vi "Que_Build Initialize Command Set.vi"(8 "Error":errorcluster, 11 "Icon Source Is From A VI":bool) -> (0 "Error Out":errorcluster, 3 "Command Set Out":T1[](array[typedef]))   [LabVIEW 2009]
doc: "Builds the Initialize command set for the producer consumer loop"
uses:
  Controls/Cluster/Cluster_Icon Fixer Command Data Set.ctl
  Controls/Enum/ENUM_Icon Fixer Commands.ctl
  Controls/Enum/ENUM_Clear Text Select.ctl
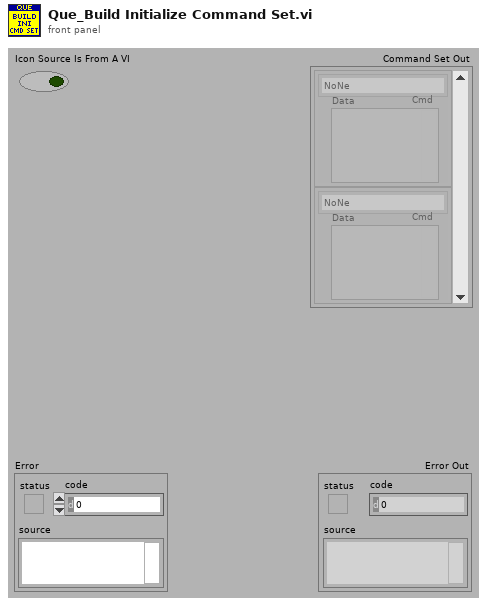
[diagram p1: front panel]
types:
  T1 = typedef "Cluster_Icon Fixer Command Data Set.ctl" = cluster{"Cmd":T2, "Data":variant}
  T2 = typedef "ENUM_Icon Fixer Commands.ctl" = enum16{"NoNe", "Initialize", "Get VI", "Extract Icon", "ReDraw New Icon", "Set Vis Icon", "Save Vi", "Clear String controls", "Set Icon Cluster", "Reset Vis Icon", "Pick Colors", "Upload icon templates", "Download icon templates", "Stop Program", "OCR", "Display Set", "Set Focus", "Set Colors"}
  T3 = typedef "ENUM_Clear Text Select.ctl" = enum16{"NoNe", "All", "Header", "Body"}
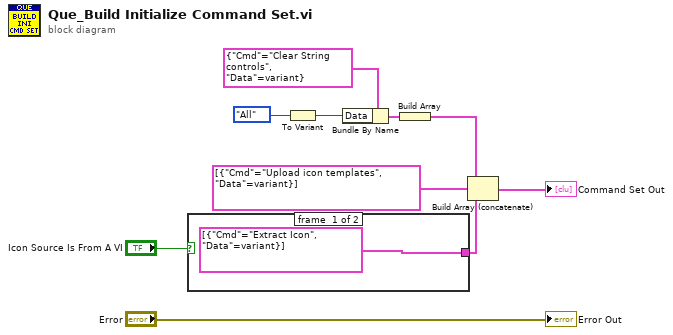
[diagram p0: block diagram]
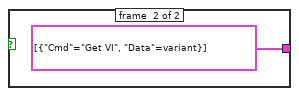
[diagram p2: hidden frame]
diagram:
  n1 = case shown="False" "Icon Source Is From A VI" {
    tunnel: [T1[] [{"Cmd"=enum."Extract Icon", "Data"=variant}] T1[] [{"Cmd"=enum."Get VI", "Data"=variant}]] -> w4
    frame #0 {
    }
    frame #1 {
    }
  }
  n2 = To Variant(anything=ENUM_Clear_Text_Select."All" ("Clear Text Select")) -> (Variant=w10:variant)
  n3 = Bundle By Name(cluster=T1 {"Cmd"=enum."Clear String controls", "Data"=variant} ("Cluster"), "Data"=w10) -> (w8:T1)
  n4 = Build Array(w8) -> (w6:T1[])
  n5 = Build Array (concatenate)(w6, T1[] [{"Cmd"=enum."Upload icon templates", "Data"=variant}] ("array"), w4) -> (→"Command Set Out":T1[])
  "Error Out" <- "Error"
